vi "Ballard 429 - Initialize.vi"(7 "RT Config Filepath":path, 8 "Error (in)":errorcluster, 11 "Card Parameters (in)":T1) -> (0 "Error (out)":errorcluster, 3 "Card Parameters (out)":T1)   [LabVIEW 2020, in "Ballard Arinc-429 Engine.lvlib"]
doc: "Arinc-429 Board Initialization."
uses:
  Ballard Arinc-429 Engine.lvlib
  RT Controls/Card Parameters.ctl
  Shared/Controls and Global/Initialization Method.ctl
  <instrlib>/BTICardLib/Private/Initialize By Card Number and Core Number.vi
  <instrlib>/BTICardLib/Private/Initialize By Slot Number and Core Number.vi
  <instrlib>/BTICardLib/Private/IO/Action-Status/Write External LED.vi
  <instrlib>/BTICardLib/Private/Configure All From XML.vi
  <instrlib>/BTI429Lib/Private/Core/Action-Status/Start All Channels.vi
  <instrlib>/BTICardLib/BTICardLV.lvlib
  <instrlib>/BTI429Lib/BTI429LV.lvlib
  Shared/Ballard Arinc-429 Shared.lvlib
  <vilib>/NI VeriStand/Custom Device Tools/Custom Device Utility Library/Custom Device Utility Library.lvlib
panel:
  out "Card Type":string
  out "Product String":string
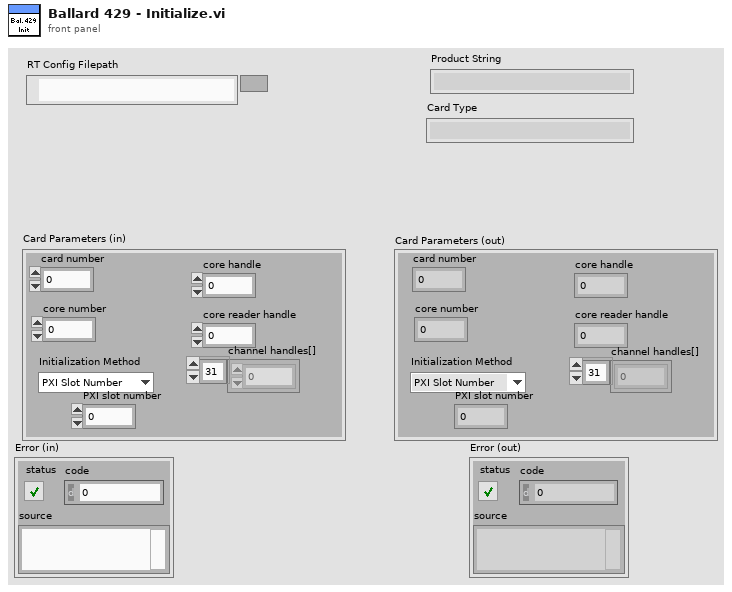
[diagram p1: front panel]
types:
  T1 = typedef "Ballard Arinc-429 Engine.lvlib/Card Parameters.ctl" = cluster{"card number":i32, "core number":i32, "core handle":u64, "core reader handle":u64, "channel handles[]":u64[], "Initialization Method":T2, "PXI slot number":i32}
  T2 = typedef "Ballard Arinc-429 Shared.lvlib/Initialization Method.ctl" = enum16{"PXI Slot Number", "Card Number"}
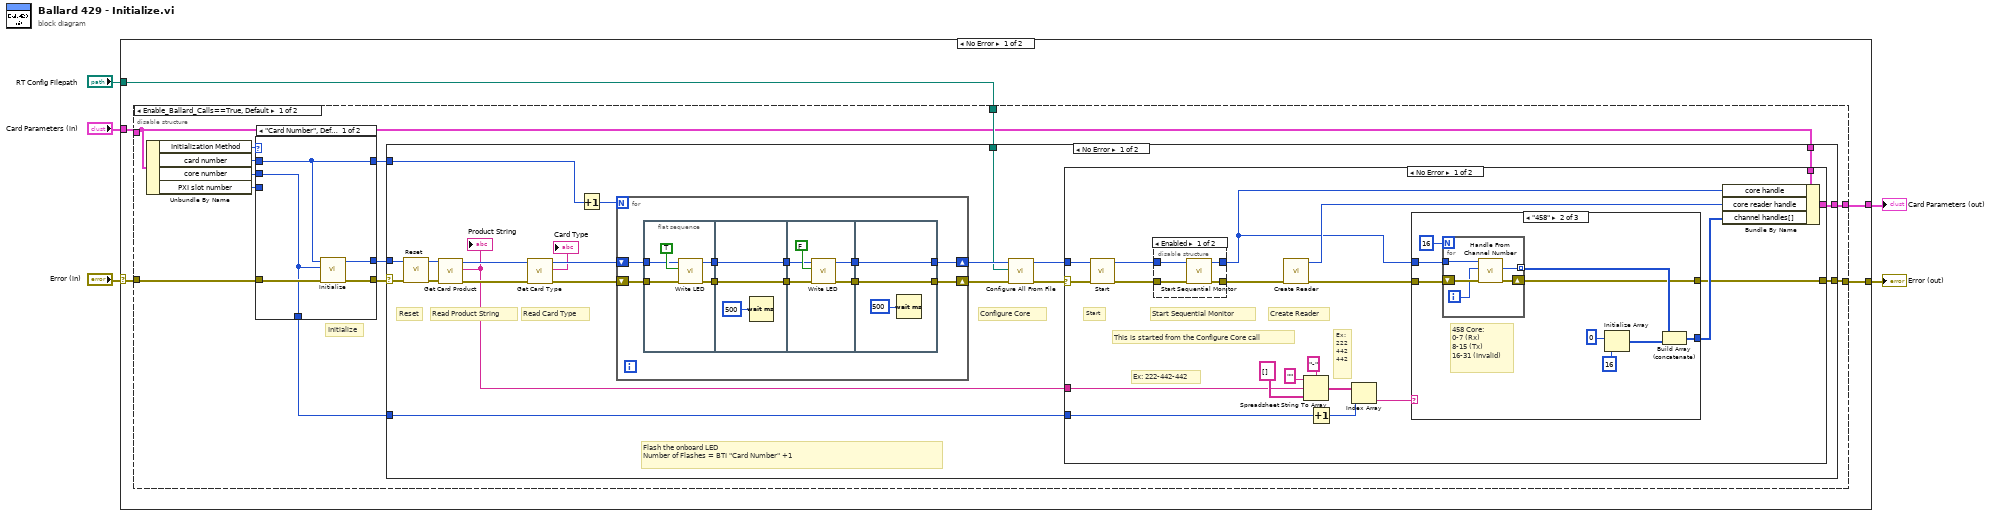
[diagram p0: block diagram]
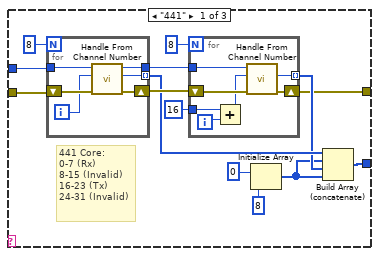
[diagram p2: hidden frame]
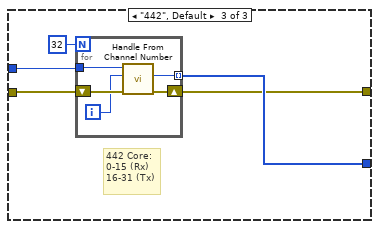
[diagram p3: hidden frame]
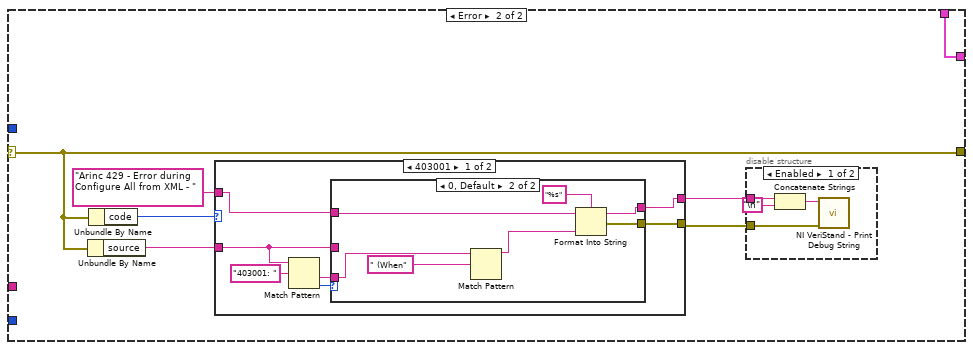
[diagram p5: hidden frame]
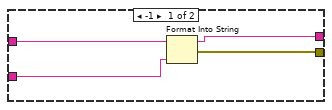
[diagram p7: hidden frame]
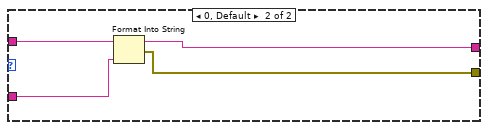
[diagram p8: hidden frame]
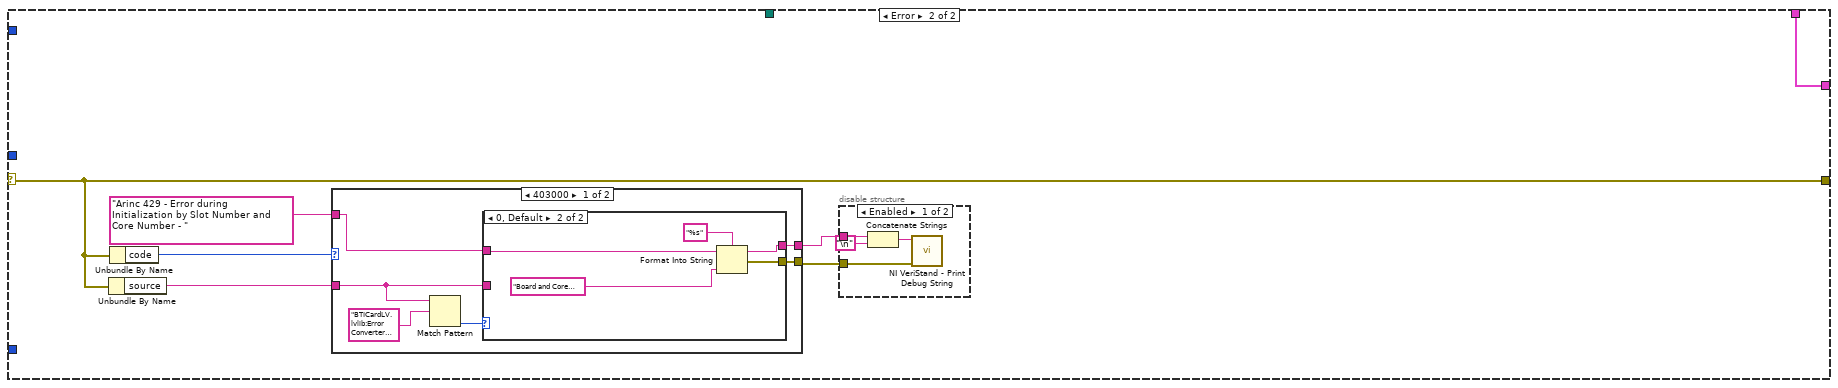
[diagram p9: hidden frame]
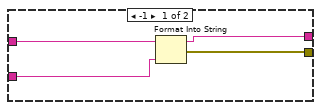
[diagram p11: hidden frame]
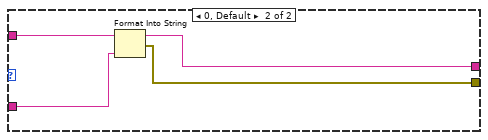
[diagram p12: hidden frame]
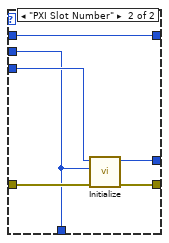
[diagram p13: hidden frame]
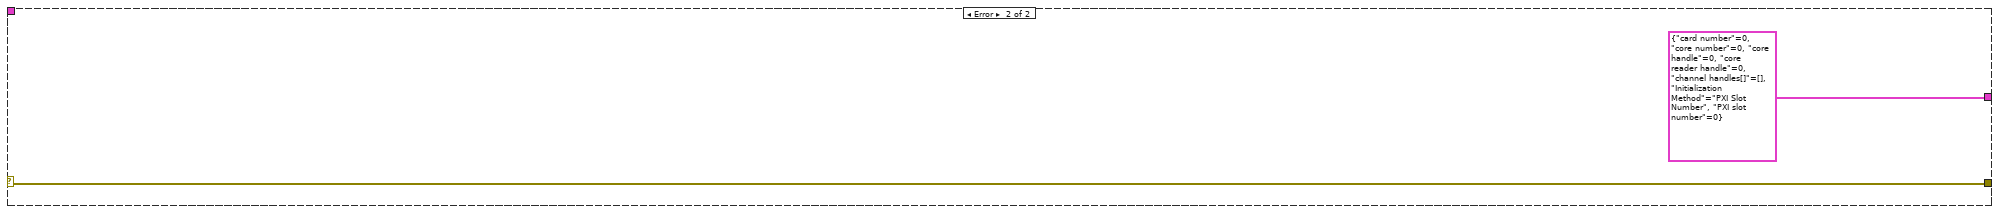
[diagram p15: hidden frame]
diagram:
  n1 = case shown="No Error" "Error (in)" {
    selector: "Error (in)" -> [w7 w225]
    tunnel: [w10 T1 {"card number"=0, "core number"=0, "core handle"=0, "core reader handle"=0, "channel handles[]"=[], "Initialization Method"=enum."PXI Slot Number", "PXI slot number"=0} ("Card Parameters (in)")] -> w5
    tunnel: "RT Config Filepath" -> [w9 _]
    tunnel: [w8 w225] -> w3
    tunnel: "Card Parameters (in)" -> [w6 _]
    frame No Error {
      n2 = disable-structure shown="Enable_Ballard_Calls==True, Default" {
        disable-tunnel: [w22 w222] -> w10
        disable-tunnel: w9 -> [w21 _]
        disable-tunnel: [w14 w223] -> w8
        disable-tunnel: w7 -> [w20 w223]
        disable-tunnel: w6 -> [w19 w222]
        frame condition #0 (active) {
          # "Initialize"
          n3 = Unbundle By Name(w19) -> ("Initialization Method"=w18:T2, "card number"=w17:i32, "core number"=w16:i32, "PXI slot number"=w15:i32)
          n4 = case shown="\"Card Number\", Default" w18 {
            tunnel: [w215 w221] -> w23
            tunnel: [w214 w220] -> w13
            tunnel: w17 -> [w212 w217]
            tunnel: w20 -> [w213 w219]
            tunnel: w16 -> [w211 w216]
            tunnel: w15 -> [_ w218]
            tunnel: [w212 w217] -> w12
            tunnel: [w211 w216] -> w11
            frame "Card Number", Default {
              n5 = call-poly <instrlib>:"Initialize.vi"("error in (no error)"=w213, "core number"=w211, "card number"=w212) -> ("error out"=w214:errorcluster, "core handle out"=w215:u64)  [unwired: 7 in]
            }
            frame "PXI Slot Number" {
              n6 = call-poly <instrlib>:"Initialize.vi"("error in (no error)"=w219, "core number"=w216, "slot number"=w218) -> ("error out"=w220:errorcluster, "core handle out"=w221:u64)  [unwired: 7 in]
            }
          }
          n7 = case shown="No Error" w13 {
            selector: w13 -> [w28 w184]
            tunnel: w23 -> [w44 _]
            tunnel: [w43 w187] -> w22
            tunnel: w21 -> [w32 _]
            tunnel: w19 -> [w31 w187]
            tunnel: w12 -> [w30 _]
            tunnel: [w29 w184] -> w14
            tunnel: w11 -> [w24 _]
            frame No Error {
              # "Configure Core"
              # "Flash the onboard LED\nNumber of Flashes = BTI \"Card Number\" +1"
              # "Read Card Type"
              # "Read Product String"
              # "Reset"
              n8 = call <instrlib>:"Reset.vi"("error in (no error)"=w28, "core handle in"=w44) -> ("error out"=w39:errorcluster, "core handle out"=w40:u64)  [unwired: 8 in]
              n9 = call <instrlib>:"Get Card Product.vi"("error in (no error)"=w39, "core handle in"=w40) -> ("error out"=w41:errorcluster, "product string out"=w25:string, "core handle out"=w42:u64)  [unwired: 7 in]
              "Product String" <- w25
              n10 = call <instrlib>:"Get Card Type.vi"("error in (no error)"=w41, "core handle in"=w42) -> ("error out"=w37:errorcluster, "type string out"=→"Card Type":string, "core handle out"=w38:u64)  [unwired: 7 in]
              n11 = Increment(x=w30) -> (x+1=w34:i32)
              n12 = for {
                N: w34 -> [_]
                shift-right: [w156] -> w36
                shift-left: w38 -> [w158]
                shift-right: [w155] -> w35
                shift-left: w37 -> [w157]
                n13 = flat-sequence {
                  tunnel: [w168] -> w164
                  tunnel: [w167] -> w163
                  tunnel: w158 -> [w166]
                  tunnel: w157 -> [w165]
                  tunnel: [w171] -> w162
                  tunnel: w164 -> [w171]
                  tunnel: [w170] -> w161
                  tunnel: w163 -> [w170]
                  tunnel: w162 -> [w176]
                  tunnel: [w175] -> w160
                  tunnel: [w174] -> w159
                  tunnel: w161 -> [w173]
                  tunnel: [w179] -> w155
                  tunnel: w160 -> [w179]
                  tunnel: [w178] -> w156
                  tunnel: w159 -> [w178]
                  frame #0 {
                    n14 = call-poly <instrlib>:"Write LED.vi"("error in (no error)"=w165, "LED state"=TRUE, "core handle in"=w166) -> ("error out"=w168:errorcluster, "core handle out"=w167:u64)  [unwired: 7 in]
                  }
                  frame #1 {
                    n15 = Wait (ms)(milliseconds to wait=u32 500) -> ()  [unwired: 1 out]
                  }
                  frame #2 {
                    n16 = call-poly <instrlib>:"Write LED.vi"("error in (no error)"=w176, "LED state"=FALSE, "core handle in"=w173) -> ("error out"=w175:errorcluster, "core handle out"=w174:u64)  [unwired: 7 in]
                  }
                  frame #3 {
                    n17 = Wait (ms)(milliseconds to wait=u32 500) -> ()  [unwired: 1 out]
                  }
                }
              }
              n18 = call-poly <instrlib>:"Configure All From File.vi"("error in (no error)"=w35, "configuration file path"=w32, "core handle in"=w36) -> ("error out"=w27:errorcluster, "core handle out"=w33:u64)  [unwired: 7 in]
              n19 = case shown="No Error" w27 {
                selector: w27 -> [w56 w123]
                tunnel: [w64 w122] -> w43
                tunnel: w33 -> [w63 _]
                tunnel: w31 -> [w59 w122]
                tunnel: [w57 w123] -> w29
                tunnel: w25 -> [w50 _]
                tunnel: w24 -> [w49 _]
                frame No Error {
                  # "Ex:\n222\n442\n442"
                  # "Ex: 222-442-442"
                  # "This is started from the Configure Core call"
                  # "Start"
                  # "Start Sequential Monitor"
                  # "Create Reader"
                  n20 = call-poly <instrlib>:"Start.vi"("error in (no error)"=w56, "core handle in"=w63) -> ("error out"=w61:errorcluster, "core handle out"=w62:u64)  [unwired: 8 in]
                  n21 = disable-structure shown="Enabled" {
                    disable-tunnel: w62 -> [w119 w121]
                    disable-tunnel: w61 -> [w118 w120]
                    disable-tunnel: [w117 w120] -> w60
                    disable-tunnel: [w116 w121] -> w45
                    frame Enabled {
                      n22 = call <instrlib>:"Start Sequential Monitor.vi"("error in (no error)"=w118, "core handle in"=w119) -> ("error out"=w117:errorcluster, "core handle out"=w116:u64)  [unwired: 8 in]
                    }
                    frame Disabled {
                    }
                  }
                  n23 = call <instrlib>:"Create Reader.vi"("error in (no error)"=w60) -> ("error out"=w55:errorcluster, "core reader handle out"=w54:u64)  [unwired: 9 in]
                  n24 = Spreadsheet String To Array(delimiter (Tab)="-", format string="", spreadsheet string=w50, array type (2D Dbl)=string[] []) -> (array=w48:string[])
                  n25 = Increment(x=w49) -> (x+1=w47:i32)
                  n26 = Index Array(array=w48, index=w47) -> (element=w46:string)
                  n27 = case shown="\"458\"" w46 {
                    tunnel: w55 -> [w77 w99 w109]
                    tunnel: w45 -> [w76 w98 w108]
                    tunnel: [w69 w94 w107] -> w58
                    tunnel: [w66 w92 w106] -> w57
                    frame "441" {
                      # "441 Core:\n0-7 (Rx)\n8-15 (Invalid)\n16-23 (Tx)\n24-31 (Invalid)"
                      n28 = for {
                        N: 8 -> [_]
                        shift-right: [w88] -> w74
                        shift-left: w77 -> [w91]
                        tunnel: [w89] -> w70 mode=indexing
                        tunnel: w76 -> [w87]
                        tunnel: [w86] -> w73
                        i -> [w90]
                        n29 = call <instrlib>:"Handle From Channel Number.vi"("error in (no error)"=w91, "channel number"=w90, "core handle in"=w87) -> ("error out"=w88:errorcluster, "channel handle out"=w89:u64, "core handle out"=w86:u64)  [unwired: 6 in]
                      }
                      n30 = for {
                        N: 8 -> [_]
                        shift-right: [w83] -> w66
                        shift-left: w74 -> [w85]
                        tunnel: [w84] -> w68 mode=indexing
                        tunnel: w73 -> [w82]
                        tunnel: 16 ("channel handle out") -> [w79]
                        i -> [w80]
                        n31 = Add(x=w79, y=w80) -> (x+y=w81:i32)
                        n32 = call <instrlib>:"Handle From Channel Number.vi"("error in (no error)"=w85, "channel number"=w81, "core handle in"=w82) -> ("error out"=w83:errorcluster, "channel handle out"=w84:u64)  [unwired: 6 in, 1 out]
                      }
                      n33 = Initialize Array(u64 0 ("channel handle out"), 8 ("dimension size")) -> (w67:u64[])
                      n34 = Build Array (concatenate)(w70, w67, w68, w67) -> (w69:u64[])
                    }
                    frame "458" {
                      # "458 Core:\n0-7 (Rx)\n8-15 (Tx)\n16-31 (Invalid)"
                      n35 = for {
                        N: 16 -> [_]
                        shift-right: [w102] -> w92
                        shift-left: w99 -> [w105]
                        tunnel: [w103] -> w95 mode=indexing
                        tunnel: w98 -> [w101]
                        i -> [w104]
                        n36 = call <instrlib>:"Handle From Channel Number.vi"("error in (no error)"=w105, "channel number"=w104, "core handle in"=w101) -> ("error out"=w102:errorcluster, "channel handle out"=w103:u64)  [unwired: 6 in, 1 out]
                      }
                      n37 = Initialize Array(u64 0 ("channel handle out"), 16 ("dimension size")) -> (w93:u64[])
                      n38 = Build Array (concatenate)(w95, w93) -> (w94:u64[])
                    }
                    frame "442", Default {
                      # "442 Core:\n0-15 (Rx)\n16-31 (Tx)"
                      n39 = for {
                        N: 32 -> [_]
                        shift-right: [w112] -> w106
                        shift-left: w109 -> [w115]
                        tunnel: [w113] -> w107 mode=indexing
                        tunnel: w108 -> [w111]
                        i -> [w114]
                        n40 = call <instrlib>:"Handle From Channel Number.vi"("error in (no error)"=w115, "channel number"=w114, "core handle in"=w111) -> ("error out"=w112:errorcluster, "channel handle out"=w113:u64)  [unwired: 6 in, 1 out]
                      }
                    }
                  }
                  n41 = Bundle By Name(cluster=w59, "core handle"=w45, "core reader handle"=w54, "channel handles[]"=w58) -> (w64:T1)
                }
                frame Error {
                  n42 = Unbundle By Name(w123) -> ("source"=w126:string)
                  n43 = Unbundle By Name(w123) -> ("code"=w124:i32)
                  n44 = case shown="403001" w124 {
                    tunnel: [w139 w152] -> w128
                    tunnel: [w138 w151] -> w127
                    tunnel: "Arinc 429 - Error during Configure All from XML - " ("String to write") -> [w136 w154]
                    tunnel: w126 -> [w137 w153]
                    frame 403001 {
                      n45 = Match Pattern(string=w137, regular expression="403001: ") -> (after substring=w133:string, offset past match=w135:i32)  [unwired: 1 in, 2 out]
                      n46 = case shown="0, Default" w135 {
                        tunnel: [w140 w150] -> w139
                        tunnel: [w141 w149] -> w138
                        tunnel: w137 -> [w142 _]
                        tunnel: w136 -> [w143 w148]
                        tunnel: w133 -> [_ w146]
                        frame -1 {
                          n47 = Format Into String(initial string=w143, w142) -> (resulting string=w140:string, error out=w141:errorcluster)  [unwired: 2 in]
                        }
                        frame 0, Default {
                          n48 = Match Pattern(string=w146, regular expression=" (When") -> (before substring=w145:string)  [unwired: 1 in, 3 out]
                          n49 = Format Into String(format string="%s", initial string=w148, w145) -> (resulting string=w150:string, error out=w149:errorcluster)  [unwired: 1 in]
                        }
                      }
                    }
                    frame 0, Default {
                      n50 = Format Into String(initial string=w154, w153) -> (resulting string=w152:string, error out=w151:errorcluster)  [unwired: 2 in]
                    }
                  }
                  n51 = disable-structure shown="Enabled" {
                    disable-tunnel: w127 -> [w130 _]
                    disable-tunnel: w128 -> [w129 _]
                    frame Enabled {
                      n52 = Concatenate Strings(w129, "\n") -> (w131:string)
                      n53 = call <vilib>:"NI VeriStand - Print Debug String.vi"("error in (no error)"=w130, "Message"=w131) -> ()  [unwired: 9 in, 1 out]
                    }
                    frame Disabled {
                    }
                  }
                }
              }
            }
            frame Error {
              n54 = Unbundle By Name(w184) -> ("source"=w183:string)
              n55 = Unbundle By Name(w184) -> ("code"=w186:i32)
              n56 = case shown="403000" w186 {
                tunnel: [w197 w208] -> w181
                tunnel: [w196 w207] -> w182
                tunnel: "Arinc 429 - Error during Initialization by Slot Number and Core Number - " ("String to write") -> [w192 w210]
                tunnel: w183 -> [w193 w209]
                frame 403000 {
                  n57 = Match Pattern(string=w193, regular expression="BTICardLV.lvlib:Error Converter (ErrCode or Status).vi<ERR>\nEncountered library error 403000=ERRTYPE_INITIALIZE Failed to initialize the card or core (LabVIEW Library)\nDebug Info: No matching slot number was found in BTICardLV_InitializeBySlotNumber.") -> (offset past match=w194:i32)  [unwired: 1 in, 3 out]
                  n58 = case shown="0, Default" w194 {
                    tunnel: [w198 w206] -> w197
                    tunnel: [w199 w205] -> w196
                    tunnel: w193 -> [w200 _]
                    tunnel: w192 -> [w201 w204]
                    frame -1 {
                      n59 = Format Into String(initial string=w201, w200) -> (resulting string=w198:string, error out=w199:errorcluster)  [unwired: 2 in]
                    }
                    frame 0, Default {
                      n60 = Format Into String(format string="%s", initial string=w204, "Board and Core combination cannot be found. Ensure Initialization method and parameters values are valid.") -> (resulting string=w206:string, error out=w205:errorcluster)  [unwired: 1 in]
                    }
                  }
                }
                frame 0, Default {
                  n61 = Format Into String(initial string=w210, w209) -> (resulting string=w208:string, error out=w207:errorcluster)  [unwired: 2 in]
                }
              }
              n62 = disable-structure shown="Enabled" {
                disable-tunnel: w182 -> [w189 _]
                disable-tunnel: w181 -> [w188 _]
                frame Enabled {
                  n63 = Concatenate Strings(w188, "\n") -> (w190:string)
                  n64 = call <vilib>:"NI VeriStand - Print Debug String.vi"("error in (no error)"=w189, "Message"=w190) -> ()  [unwired: 9 in, 1 out]
                }
                frame Disabled {
                }
              }
            }
          }
        }
        frame condition #1 {
        }
      }
    }
    frame Error {
    }
  }
  "Error (out)" <- w3
  "Card Parameters (out)" <- w5
